vi "While-loop-sample.vi"() -> ()   [LabVIEW 2020]
panel:
  in  "stop\nloop":bool
  out "Loop\nCount":i32
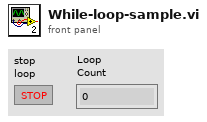
[diagram p1: front panel]
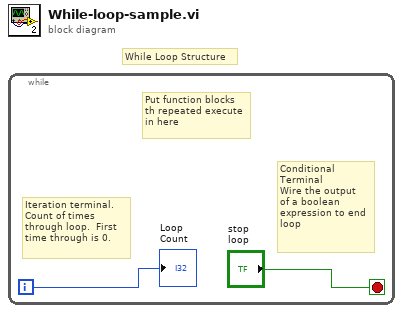
[diagram p0: block diagram]
diagram:
  # "While Loop Structure"
  n1 = while {
    i -> [w2]
    stop <- "stop\nloop" stop-if-true
    # "Put function blocks\nth repeated execute\nin here"
    # "Conditional\nTerminal\nWire the output\nof a boolean\nexpression to end\nloop"
    # "Iteration terminal.\nCount of times \nthrough loop.  First \ntime through is 0."
    "Loop\nCount" <- w2
  }
